vi "init_steps_protocol_v02.vi"(4 "sampling rate (Hz)":i32, 6 "samples to read":i32, 8 "AO error in":errorcluster, 9 "AO physical channels":tag="cDAQ1Mod3/ao14", 10 "AI error in":errorcluster, 11 "AI Physical Channel":tag="cDAQ1Mod1/ai0") -> (0 "error out":errorcluster, 1 "AO out":refnum<k21>, 3 "AI out":refnum<k21>)   [LabVIEW 2015]
uses:
  <vilib>/DAQmx/configure/timing.llb/DAQmx Timing (Sample Clock).vi
  <vilib>/DAQmx/configure/trigger.llb/DAQmx Start Trigger (Digital Edge).vi
  <vilib>/DAQmx/create/channels.llb/DAQmx Create Channel (AO-Voltage-Basic).vi
  <vilib>/DAQmx/create/channels.llb/DAQmx Create Channel (AI-Voltage-Basic).vi
panel:
  # "INIT CLAMP PROTOCOL"
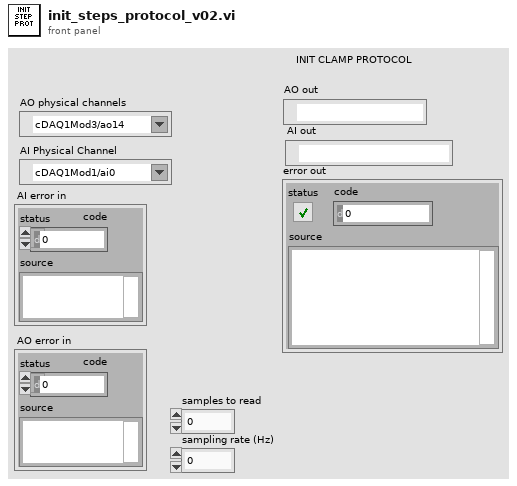
[diagram p1: front panel]
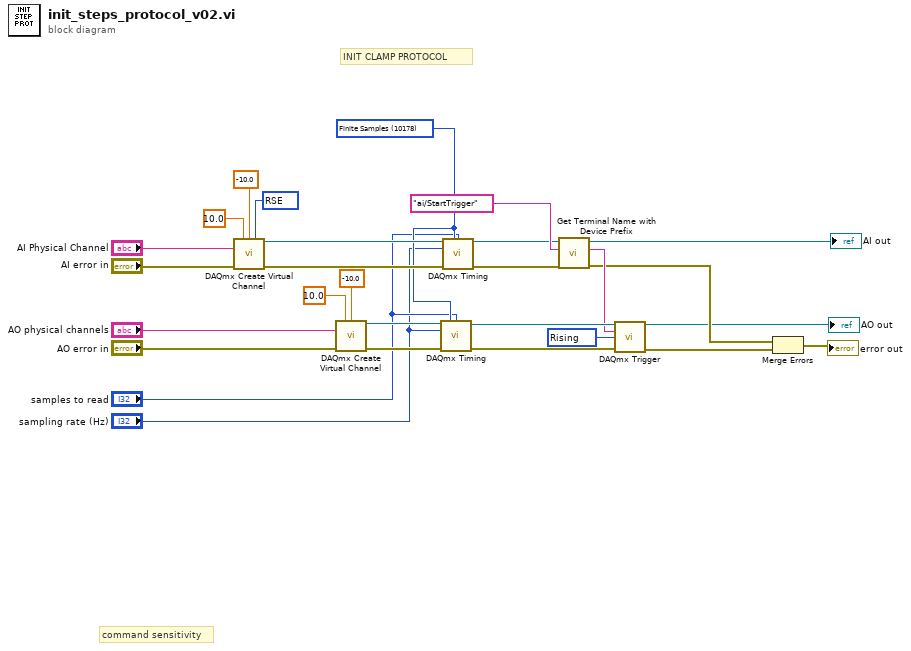
[diagram p0: block diagram]
diagram:
  w6 = 10280 items=["Rising"=10280, "Falling"=10171] ("edge")
  w25 = 10083 items=["default"=-1, "RSE"=10083, "NRSE"=10078, "Differential"=10106, "Pseudodifferential"=12529] ("input terminal configuration")
  w17 = 10178 items=["Finite Samples"=10178, "Continuous Samples"=10123] ("sample mode")
  # "INIT CLAMP PROTOCOL"
  # "command sensitivity"
  n1 = call-poly <vilib>:"DAQmx Create Virtual Channel.vi"("maximum value"=10.0, "minimum value"=-10.0, "input terminal configuration"=w25, "physical channels"="AI Physical Channel", "error in"="AI error in") -> ("task out"=w27:refnum<k21>, "error out"=w28:errorcluster)  [unwired: 9 in]
  n2 = call-poly <vilib>:"DAQmx Create Virtual Channel.vi"("maximum value"=10.0, "minimum value"=-10.0, "physical channels"="AO physical channels", "error in"="AO error in") -> ("task out"=w19:refnum<k21>, "error out"=w18:errorcluster)  [unwired: 10 in]
  n3 = call-poly <vilib>:"DAQmx Timing.vi"("task/channels in"=w19, "sample mode"=w17, "samples per channel"="samples to read", "rate"="sampling rate (Hz)", "error in"=w18) -> ("task out"=w15:refnum<k21>, "error out"=w16:errorcluster)  [unwired: 9 in]
  n4 = call-poly <vilib>:"DAQmx Timing.vi"("task/channels in"=w27, "sample mode"=w17, "samples per channel"="samples to read", "rate"="sampling rate (Hz)", "error in"=w28) -> ("task out"=w5:refnum<k21>, "error out"=w22:errorcluster)  [unwired: 9 in]
  n5 = call "Get Terminal Name with Device Prefix.vi"("error in (no error)"=w22, "Local Terminal Name"="ai/StartTrigger" ("terminal"), "task/channels in"=w5) -> ("error out"=w3:errorcluster, "Terminal Name with Device Prefix"=w14:tag, "task out"=→"AI out":refnum<k21>)  [unwired: 6 in]
  n6 = call-poly <vilib>:"DAQmx Trigger.vi"("task/channels in"=w15, "source"=w14, "edge"=w6, "error in"=w16) -> ("task out"=→"AO out":refnum<k21>, "error out"=w2:errorcluster)  [unwired: 10 in]
  n7 = Merge Errors(w3, w2) -> (→"error out":errorcluster)
